vi "sv_Modify Channel Names_Copy.vi"(7 "suffix":string=" (All)", 8 "waveforms":waveform(dbl)[](array[waveform]), 9 "prefix":string) -> (2 "renamed waveforms":waveform(dbl)[](array[waveform]))   [LabVIEW 2021, in "Audio ADC Shared.lvlib"]
doc: "Modify channel name attribute to distinguish signals in graph plot legend."
uses:
  Audio ADC Shared.lvlib
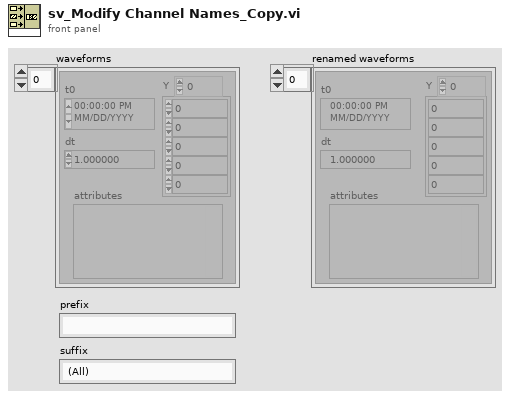
[diagram p1: front panel]
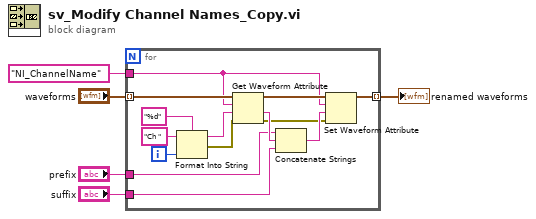
[diagram p0: block diagram]
diagram:
  n1 = for {
    tunnel: "waveforms" -> [w14] mode=indexing
    tunnel: [w13] -> w4 mode=indexing
    tunnel: "NI_ChannelName" ("name") -> [w9]
    tunnel: "suffix" -> [w8]
    tunnel: "prefix" -> [w7]
    i -> [w17]
    n2 = Format Into String(format string="%d", initial string="Ch ", w17) -> (resulting string=w12:string, error out=w6:errorcluster)  [unwired: 1 in]
    n3 = Get Waveform Attribute(4:w6, 5:w12, 6:w9, 7:w14) -> (0:w10:errorcluster, 1:w11:string, 3:w16:waveform(dbl))  [unwired: 1 out]
    n4 = Concatenate Strings(w7, w11, w8) -> (w15:string)
    n5 = Set Waveform Attribute(4:w10, 5:w15, 6:w9, 7:w16) -> (3:w13:waveform(dbl))  [unwired: 2 out]
  }
  "renamed waveforms" <- w4
